vi "Select Side.vi"(7 "Side":T1, 9 "Column":i32, 10 "Row":i32, 11 "Array in":i32[][](array[numeric])) -> (1 "Column Out":i32[](array[numeric]), 2 "Row Out":i32[](array[numeric]), 3 "Values":i32[](array[numeric]), 5 "Counter Side":T1)   [LabVIEW 2019, in "Day 15.lvlib"]
uses:
  Day 15.lvlib
  Day 11/Controls/Side.ctl
  Day 11/Day 11.lvlib
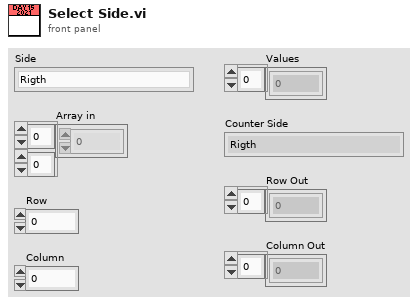
[diagram p1: front panel]
types:
  T1 = typedef "Day 11.lvlib/Side.ctl" = enum16{"Rigth", "Left", "Down", "Up", "Rigth Up", "Rigth Down", "Left Up", "Left Down"}
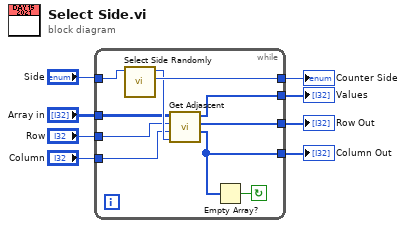
[diagram p0: block diagram]
diagram:
  n1 = while {
    tunnel: [w15] -> w6
    tunnel: "Array in" -> [w14]
    tunnel: [w10] -> w4
    tunnel: [w13] -> w3
    tunnel: "Column" -> [w12]
    tunnel: "Row" -> [w11]
    tunnel: "Side" -> [w17]
    tunnel: [w18] -> w8
    stop <- w9 continue-if-true
    n2 = call "Select Side Randomly.vi"("Do not include this side"=w17) -> ("Counter Side"=w18:T1, "Side"=w16:T1)  [unwired: 9 in]
    n3 = call "Get Adjascent.vi"("Side"=w16, "Column In"=w12, "Row In"=w11, "Array In"=w14) -> ("Column Out"=w10:i32[], "Row Out"=w13:i32[], "Array"=w15:i32[])  [unwired: 5 in]
    n4 = Empty Array?(array=w10) -> (empty?=w9:bool)
  }
  "Counter Side" <- w8
  "Values" <- w6
  "Column Out" <- w4
  "Row Out" <- w3
